vi "Continuous.vi"(8 "error in":errorcluster, 10 "Interval (0)":dbl min=0.0 max=99999999.0 step=0.1 format="%#_10f", 11 "VISA resource name":refnum<visa-resource-name>) -> (0 "error out":errorcluster, 3 "VISA resource name out":refnum<visa-resource-name>)   [LabVIEW 2016, in "Andeen-Hagerling 2550.lvlib"]
doc: "This VI initiates or halts continuous capacitance measurement by the bridge. The interval parameter represents the start of one measurement to the start of the next."
uses:
  Andeen-Hagerling 2550.lvlib
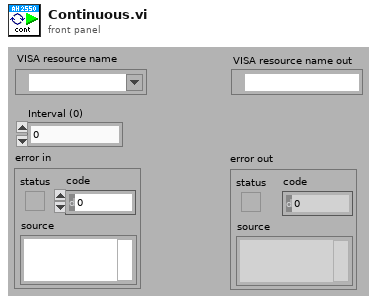
[diagram p1: front panel]
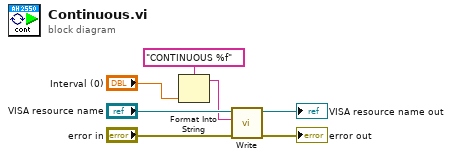
[diagram p0: block diagram]
diagram:
  n1 = Format Into String(format string="CONTINUOUS %f", "Interval (0)") -> (resulting string=w2:string)  [unwired: 2 in, 1 out]
  n2 = call "Write.vi"("error in"="error in", "command"=w2, "VISA resource name"="VISA resource name") -> ("error out"=→"error out":errorcluster, "VISA resource name out"=→"VISA resource name out":refnum<visa-resource-name>)  [unwired: 7 in]
